vi "Set_V_III.vi"(0 "Se bubbler":T1={"Dilution"=FALSE, "Calculated"=0, "MFC1 flow"=0.0, "MFC2 flow"=10.0, "MFC3 flow"=100.0, "Main"={"Flow"=0.0, "Prep"=FALSE, "Run"=FALSE, "Active"=FALSE, "Name"=""}} {"Main"."Flow" format="%.2f"; "MFC1 flow" format="%.4f"; "MFC3 flow" format="%.1f"; "MFC2 flow" format="%.2f"; "Calculated" items=["Flow", "MFC1", "MFC2", "MFC3"]}, 1 "P bubbler":T2 {"Flow" format="%.2f"}, 2 "As gas":T2 {"Flow" format="%.2f"}, 3 "P gas":T2 {"Flow" format="%.2f"}, 6 "Run Started":bool, 8 "Zn bubbler":T1={"Dilution"=FALSE, "Calculated"=0, "MFC1 flow"=0.0, "MFC2 flow"=10.0, "MFC3 flow"=100.0, "Main"={"Flow"=0.0, "Prep"=FALSE, "Run"=FALSE, "Active"=FALSE, "Name"=""}} {"Main"."Flow" format="%.2f"; "MFC1 flow" format="%.4f"; "MFC3 flow" format="%.1f"; "MFC2 flow" format="%.2f"; "Calculated" items=["Flow", "MFC1", "MFC2", "MFC3"]}, 9 "In bubbler":T2 {"Flow" format="%.2f"}, 10 "Ga bubbler":T1={"Dilution"=FALSE, "Calculated"=0, "MFC1 flow"=0.0, "MFC2 flow"=10.0, "MFC3 flow"=100.0, "Main"={"Flow"=0.0, "Prep"=FALSE, "Run"=FALSE, "Active"=FALSE, "Name"=""}} {"Main"."Flow" format="%.2f"; "MFC1 flow" format="%.4f"; "MFC3 flow" format="%.1f"; "MFC2 flow" format="%.2f"; "Calculated" items=["Flow", "MFC1", "MFC2", "MFC3"]}, 11 "Al bubbler":T2 {"Flow" format="%.2f"}) -> ()   [LabVIEW 2011]
uses:
  source_noDilution.ctl
  source_dilution.ctl
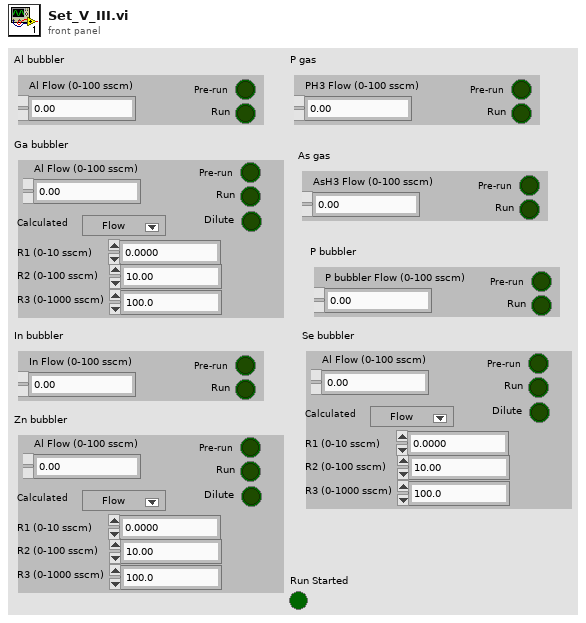
[diagram p1: front panel]
types:
  T1 = typedef "source_dilution.ctl" = cluster{"Dilution":bool, "Calculated":u16, "MFC1 flow":dbl, "MFC2 flow":dbl, "MFC3 flow":dbl, "Main":T2}
  T2 = typedef "source_noDilution.ctl" = cluster{"Flow":dbl, "Prep":bool, "Run":bool, "Active":bool, "Name":string}
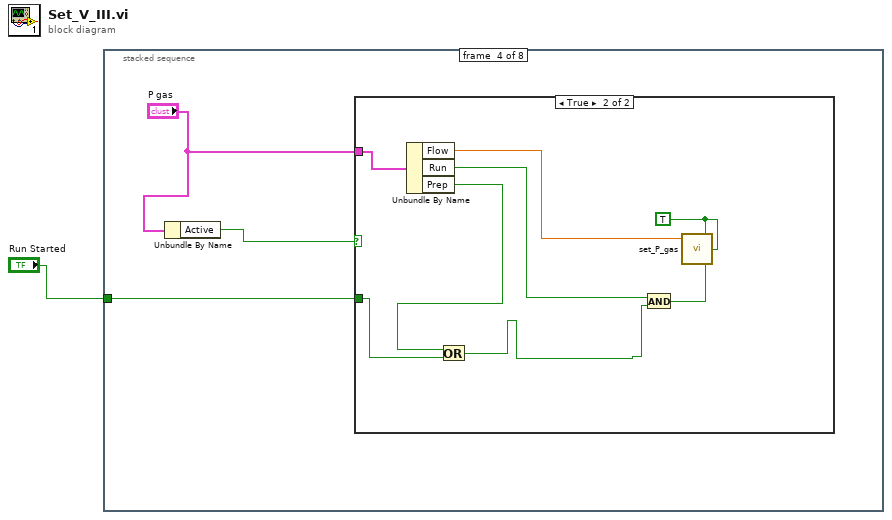
[diagram p0: block diagram]
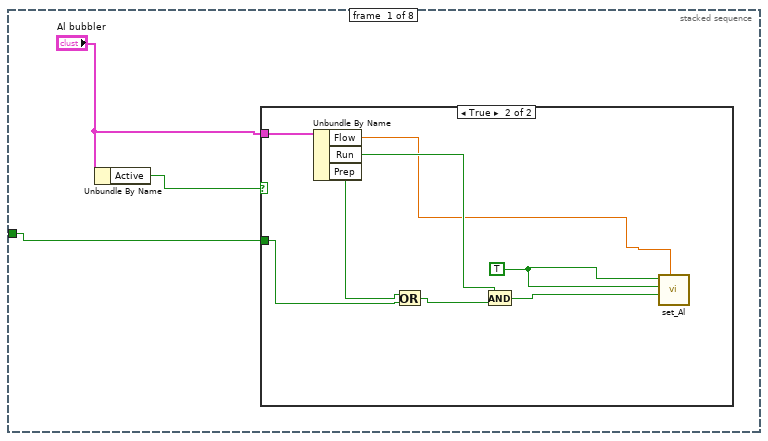
[diagram p2: hidden frame]
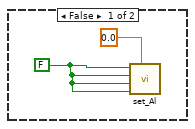
[diagram p3: hidden frame]
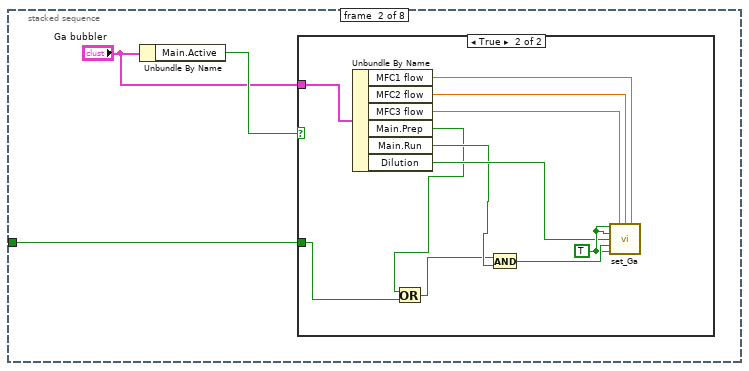
[diagram p4: hidden frame]
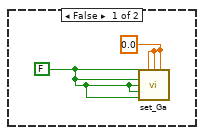
[diagram p5: hidden frame]
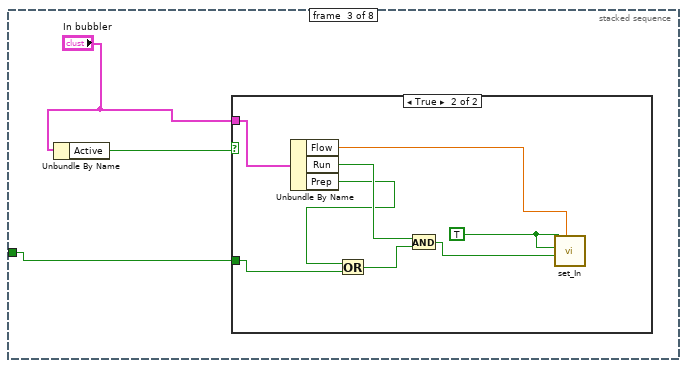
[diagram p6: hidden frame]
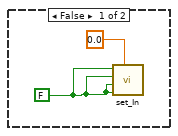
[diagram p7: hidden frame]
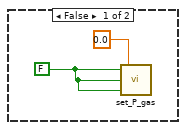
[diagram p8: hidden frame]
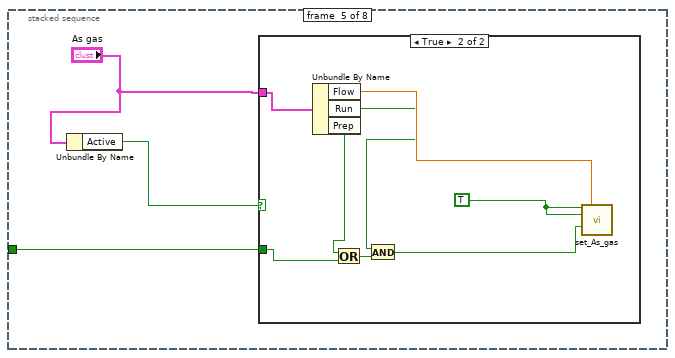
[diagram p9: hidden frame]
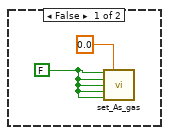
[diagram p10: hidden frame]
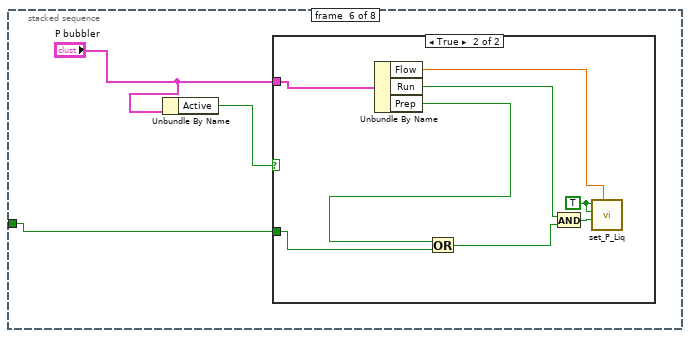
[diagram p11: hidden frame]
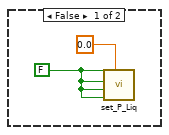
[diagram p12: hidden frame]
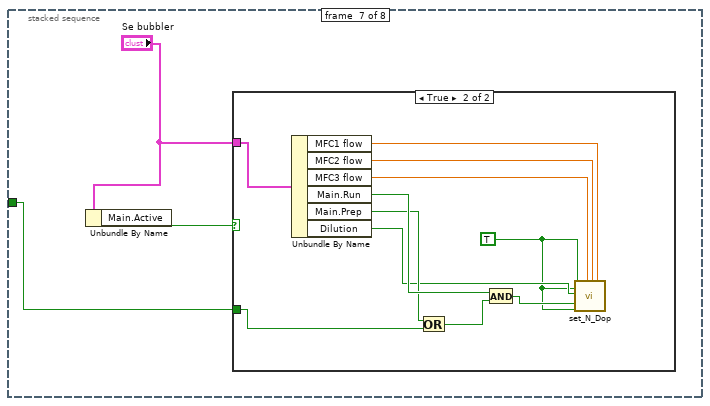
[diagram p13: hidden frame]
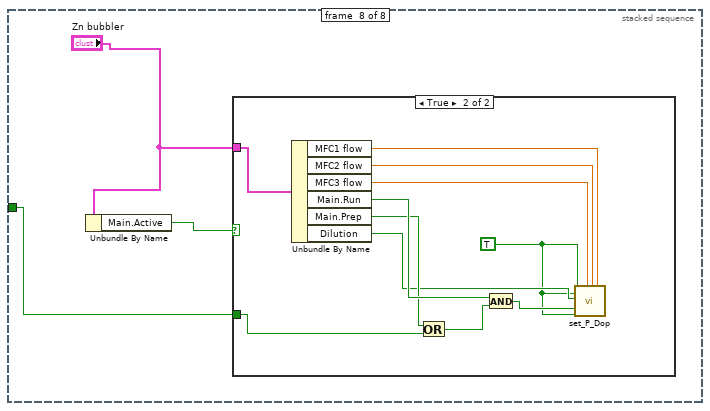
[diagram p15: hidden frame]
diagram:
  n1 = stacked-sequence {
    tunnel: "Run Started" -> [w2 w15 w31 w44 w57 w70 w83 w99]
    frame #0 {
      n2 = Unbundle By Name("Al bubbler") -> ("Active"=w4:bool)
      n3 = case shown="True" w4 {
        tunnel: "Al bubbler" -> [_ w12]
        tunnel: w2 -> [_ w8]
        frame False {
          w5 = FALSE ("Al Active")
          n4 = call "set_Al.vi"("ALMFC1"=0.0 ("Aluminum Flow"), "Remote"=w5, "Run"=w5, "Bubbler In"=w5, "Active"=w5) -> ()  [unwired: 5 out]
        }
        frame True {
          w14 = TRUE ("Al Active")
          n5 = Unbundle By Name(w12) -> ("Flow"=w10:dbl, "Run"=w11:bool, "Prep"=w9:bool)
          n6 = Or(x=w9, y=w8) -> (x .or. y?=w7:bool)
          n7 = And(x=w11, y=w7) -> (x .and. y?=w13:bool)
          n8 = call "set_Al.vi"("ALMFC1"=w10, "Run"=w13, "Bubbler In"=w14, "Active"=w14) -> ()  [unwired: 1 in, 5 out]
        }
      }
    }
    frame #1 {
      n9 = Unbundle By Name("Ga bubbler") -> ("Main.Active"=w17:bool)
      n10 = case shown="True" w17 {
        tunnel: "Ga bubbler" -> [_ w28]
        tunnel: w15 -> [_ w22]
        frame False {
          w19 = FALSE ("Ga Active")
          w18 = 0.0 ("Ga Flow 1")
          n11 = call "set_Ga.vi"("Active"=w19, "GAMFC3"=w18, "GAMFC2"=w18, "GAMFC1"=w18, "Bubbler In"=w19, "H2 Dilute"=w19, "Run"=w19, "Remote"=w19) -> ()  [unwired: 8 out]
        }
        frame True {
          w29 = TRUE ("Ga Active")
          n12 = Unbundle By Name(w28) -> ("MFC1 flow"=w27:dbl, "MFC2 flow"=w26:dbl, "MFC3 flow"=w25:dbl, "Main.Prep"=w21:bool, "Main.Run"=w23:bool, "Dilution"=w24:bool)
          n13 = Or(x=w21, y=w22) -> (x .or. y?=w20:bool)
          n14 = And(x=w20, y=w23) -> (x .and. y?=w30:bool)
          n15 = call "set_Ga.vi"("Active"=w29, "GAMFC3"=w25, "GAMFC2"=w26, "GAMFC1"=w27, "Bubbler In"=w29, "H2 Dilute"=w24, "Run"=w30, "Remote"=w29) -> ()  [unwired: 8 in]
        }
      }
    }
    frame #2 {
      n16 = Unbundle By Name("In bubbler") -> ("Active"=w33:bool)
      n17 = case shown="True" w33 {
        tunnel: "In bubbler" -> [_ w41]
        tunnel: w31 -> [_ w38]
        frame False {
          w35 = FALSE ("In Remote")
          n18 = call "set_In.vi"("INMFC1"=0.0 ("Indium Flow"), "Remote"=w35, "Run"=w35, "Bubbler In"=w35, "Active"=w35) -> ()  [unwired: 5 out]
        }
        frame True {
          w43 = TRUE ("In Run")
          n19 = Unbundle By Name(w41) -> ("Flow"=w40:dbl, "Run"=w39:bool, "Prep"=w37:bool)
          n20 = Or(x=w37, y=w38) -> (x .or. y?=w36:bool)
          n21 = And(x=w39, y=w36) -> (x .and. y?=w42:bool)
          n22 = call "set_In.vi"("INMFC1"=w40, "Run"=w42, "Bubbler In"=w43, "Active"=w43) -> ()  [unwired: 1 in, 5 out]
        }
      }
    }
    frame #3 {
      n23 = Unbundle By Name("P gas") -> ("Active"=w46:bool)
      n24 = case shown="True" w46 {
        tunnel: "P gas" -> [_ w56]
        tunnel: w44 -> [_ w53]
        frame False {
          w47 = FALSE ("P_Gas Active")
          n25 = call "set_P_gas.vi"("Run"=w47, "Gas In"=w47, "Active"=w47, "P_Gas Remote"=w47, "H2 Flush"=w47, "P_Gas Flow"=0.0) -> ()
        }
        frame True {
          w50 = TRUE ("P_Gas Active")
          n26 = Unbundle By Name(w56) -> ("Flow"=w55:dbl, "Run"=w54:bool, "Prep"=w52:bool)
          n27 = Or(x=w52, y=w53) -> (x .or. y?=w51:bool)
          n28 = And(x=w54, y=w51) -> (x .and. y?=w49:bool)
          n29 = call "set_P_gas.vi"("Run"=w49, "Gas In"=w50, "Active"=w50, "P_Gas Flow"=w55) -> ()  [unwired: 2 in]
        }
      }
    }
    frame #4 {
      n30 = Unbundle By Name("As gas") -> ("Active"=w59:bool)
      n31 = case shown="True" w59 {
        tunnel: "As gas" -> [_ w67]
        tunnel: w57 -> [_ w64]
        frame False {
          w60 = FALSE ("As_Gas Active")
          n32 = call "set_As_gas.vi"("Active"=w60, "As_Gas Flow"=0.0, "Gas In"=w60, "H2 Flush"=w60, "Run"=w60, "Remote"=w60) -> ()  [unwired: 10 in]
        }
        frame True {
          w69 = TRUE ("As_Gas Active")
          n33 = Unbundle By Name(w67) -> ("Flow"=w66:dbl, "Run"=w65:bool, "Prep"=w63:bool)
          n34 = Or(x=w63, y=w64) -> (x .or. y?=w62:bool)
          n35 = And(x=w65, y=w62) -> (x .and. y?=w68:bool)
          n36 = call "set_As_gas.vi"("Active"=w69, "As_Gas Flow"=w66, "Gas In"=w69, "Run"=w68) -> ()  [unwired: 12 in]
        }
      }
    }
    frame #5 {
      n37 = Unbundle By Name("P bubbler") -> ("Active"=w72:bool)
      n38 = case shown="True" w72 {
        tunnel: "P bubbler" -> [_ w80]
        tunnel: w70 -> [_ w75]
        frame False {
          w73 = FALSE ("As_Gas Active")
          n39 = call "set_P_Liq.vi"("flow 1"=0.0 ("As_Gas Flow"), "Remote"=w73, "Run"=w73, "Bubbler In"=w73, "Active"=w73) -> ()  [unwired: 5 in]
        }
        frame True {
          w82 = TRUE ("As_Gas Active")
          n40 = Unbundle By Name(w80) -> ("Flow"=w79:dbl, "Run"=w78:bool, "Prep"=w76:bool)
          n41 = Or(x=w76, y=w75) -> (x .or. y?=w77:bool)
          n42 = And(x=w78, y=w77) -> (x .and. y?=w81:bool)
          n43 = call "set_P_Liq.vi"("flow 1"=w79, "Run"=w81, "Bubbler In"=w82, "Active"=w82) -> ()  [unwired: 6 in]
        }
      }
    }
    frame #6 {
      n44 = Unbundle By Name("Se bubbler") -> ("Main.Active"=w85:bool)
      n45 = case shown="True" w85 {
        tunnel: "Se bubbler" -> [_ w96]
        tunnel: w83 -> [_ w90]
        frame False {
        }
        frame True {
          w86 = TRUE
          n46 = Unbundle By Name(w96) -> ("MFC1 flow"=w95:dbl, "MFC2 flow"=w94:dbl, "MFC3 flow"=w93:dbl, "Main.Run"=w92:bool, "Main.Prep"=w91:bool, "Dilution"=w88:bool)
          n47 = Or(x=w91, y=w90) -> (x .or. y?=w89:bool)
          n48 = And(x=w92, y=w89) -> (x .and. y?=w87:bool)
          n49 = call "set_N_Dop.vi"("Active"=w86, "Bubbler In"=w86, "H2 Dilute"=w88, "Run"=w87, "Remote"=w86, "Flow 3"=w93, "Flow 2"=w94, "Flow 1"=w95) -> ()  [unwired: 12 in]
        }
      }
    }
    frame #7 {
      n50 = Unbundle By Name("Zn bubbler") -> ("Main.Active"=w97:bool)
      n51 = case shown="True" w97 {
        tunnel: "Zn bubbler" -> [_ w110]
        tunnel: w99 -> [_ w104]
        frame False {
        }
        frame True {
          w100 = TRUE
          n52 = Unbundle By Name(w110) -> ("MFC1 flow"=w109:dbl, "MFC2 flow"=w108:dbl, "MFC3 flow"=w107:dbl, "Main.Run"=w106:bool, "Main.Prep"=w105:bool, "Dilution"=w102:bool)
          n53 = Or(x=w105, y=w104) -> (x .or. y?=w103:bool)
          n54 = And(x=w106, y=w103) -> (x .and. y?=w101:bool)
          n55 = call "set_P_Dop.vi"("P_Dop Active"=w100, "P_Dop Bubbler"=w100, "P_Dop H2 Dilute"=w102, "P_Dop Run"=w101, "P_Dop Remote"=w100, "P_Dop Flow 3"=w107, "P_Dop Flow 2"=w108, "P_Dop Flow 1"=w109) -> ()  [unwired: 12 in]
        }
      }
    }
  }
